vi "Drive Controller.vi"(8 "error in":errorcluster) -> ()   [LabVIEW 2018]
doc: "This VI executes continuously carrying out the current operation and responding to updates or new operation requests. It will often contain the timing or control code that is difficult to place directly in TeleOp. This VI generally opens all sensors and motors and isolates the rest of the robot code from knowing implementation details of how the operations are carried out."
uses:
  <vilib>/Rock Robotics/WPI/Framework/Completion Status.ctl
  Drive Setpoints.ctl
  Drive Operations.ctl
  Shared/RobotNeededPathData.ctl
  <vilib>/Rock Robotics/WPI/SafetyOutput/WPI_SafetyOutputConfigMenu.ctl
  <vilib>/Rock Robotics/SystemInterfaces/DIO/FPGA_DIOPWMChannel.ctl
  <vilib>/Rock Robotics/SystemInterfaces/DIO/FPGA_DIOChannel.ctl
  <vilib>/Rock Robotics/SystemInterfaces/i2clib/i2c_bus.ctl
  <vilib>/Rock Robotics/WPI/DriverStation/WPI_DriverStationRobotMode2.ctl
  <vilib>/Rock Robotics/WPI/ThirdParty/Sensors/navX/_TypeDefs/FRIC_navX_DeviceNumbersTypeDef.ctl
  <extravilib>/ChannelInstances/Lossy Stream-c(dbl,dbl,dbl,c(dbl,dbl))/Write With Abort.vi
  <extravilib>/ChannelInstances/Lossy Stream-c(dbl,dbl,dbl,c(dbl,dbl))/Read With Abort.vi
  <extravilib>/ChannelInstances/Lossy Stream-c(dbl,dbl,dbl,c(dbl,dbl))/Endpoint.vi
  <extravilib>/ChannelInstances/Lossy Stream-c(dbl,dbl,dbl,c(dbl,dbl))/EndpointRead.vi
  <vilib>/Rock Robotics/WPI/RobotDrive/WPI_RobotDriveOpen4MotorWithSPARK.vi
  <vilib>/Rock Robotics/WPI/Counter/WPI_CounterDigitalInputToDigitalSource.vi
  <vilib>/Rock Robotics/WPI/RobotDrive/WPI_RobotDriveOpen2MotorWithSPARK.vi
  Drive Published Globals.vi
  <vilib>/Rock Robotics/Network Tables/NT Write Number.vi
  <extravilib>/ChannelInstances/Lossy Stream-c(dbl,dbl,dbl,c(dbl,dbl))/Instantiate.vi
  Framework/Robot Global Data.vi
  <extravilib>/ChannelInstances/Lossy Stream-c(dbl,dbl,dbl,c(dbl,dbl))/)Channel.vi
  <resource>/ChannelSupport/_ChannelSupport/WaitIfNeeded.vi
  <vilib>/addons/control/pid/pid.llb/PID (DBL).vi
  Configuration/Constants.vi
  <vilib>/Rock Robotics/Network Tables/NT Read Number.vi
  <vilib>/addons/control/pid/NI_PID_pid.lvlib
  <extravilib>/ChannelInstances/Lossy Stream-c(dbl,dbl,dbl,c(dbl,dbl)).lvlib
panel:
  in  "Integral Range":dbl=15.0
  in  "PixyCenteringValues":cluster{"X":dbl, "Y":dbl}[](array[cluster])=[{"X"=0.0, "Y"=70.0}, {"X"=70.0, "Y"=100.0}]
  in  "EndCondArea":i32=11000
  in  "MaxY":i32=130
  in  "KpY":dbl=0.0001
  in  "KpX":dbl=0.1
  in  "MaxSpeed":dbl=0.3
  in  "KdX":dbl=0.07
  in  "AreaSetpoint":i32
  in  "CenterSetpoint":i32=80
  out "PID Tuining":cluster{dbl, dbl}(graph)={170.0, 167.02}
  in  "Points":cluster{"X":dbl, "Y":dbl}[](array[cluster])=[{"X"=0.0, "Y"=0.0}, {"X"=0.01, "Y"=0.0}, {"X"=0.011, "Y"=0.17}, {"X"=1.0, "Y"=1.0}]
  in  "PID gains":T1={"proportional gain (Kc)"=0.01, "integral time (Ti, min)"=0.007, "derivative time (Td, min)"=0.0015} {"derivative time (Td, min)" format="%#_9g"}
  out "Numeric":dbl=4.0
  out "Yaw 2":dbl=-45.089999999999996
  in  "Gains":T2={"FFV"=0.0059, "FFA"=0.0019, "Vel PID"={"P"=0.01, "I"=0.0, "D"=0.0}}
  in  "Interactive Values":T3={"Operation"=enum."Turn to Angle", "Left Speed"=-0.27, "Right Speed"=0.27, "Duration"=2.0, "Speed"=0.0, "Start Angle"=0.0, "Target Angle"=180.0, "Distance (inch)"=0.0, "Start Point (inch)"=0.0, "RobotNeededPathData"={"Path"=[], "MaxVel"=0.0, "MaxAccel"=-1.0, "Backwards?"=FALSE, "PointSpacing"=0.0, "LookaheadDist"=0.0, "Speed/Curve"=1.8, "SlowDistanceAtEnd"=12.0, "SlowSpeed"=15.0, "MaxDeAccel"=0.0}, "Start Point 2"=0.0} {"RobotNeededPathData"."SlowSpeed" format="%#_13g"; "RobotNeededPathData"."SlowDistanceAtEnd" format="%#_13g"; "RobotNeededPathData"."Speed/Curve" format="%#_13g"}
  in  "Buttons":cluster{"Execute Cmd":bool, "Abort Cmd":bool}
  out "Command Timing":cluster{"Start Time (ms)":u32, "Iterations":i32}={"Start Time (ms)"=372507, "Iterations"=0}
  out "Status":T6
  out "Setpoints":T7(graph)
  out "Current\nCmd":string="Started at  14:51:47.884\nDefault: Reserve,  L 0.0, R 0.0, D 0.000000"
  # "Tip: The graph shows the motor setpoints. It may also be helpful to observe inputs and sensor values.\nYou may also want to display tuning or debugging controls."
  # ".0088"
  # ".0017"
  # ".02"
  # "Interactive Command: You may fill in the settings for a command\nand schedule it with the Execute button. You can observe and abort\nany command while fine tuning the code for the controller."
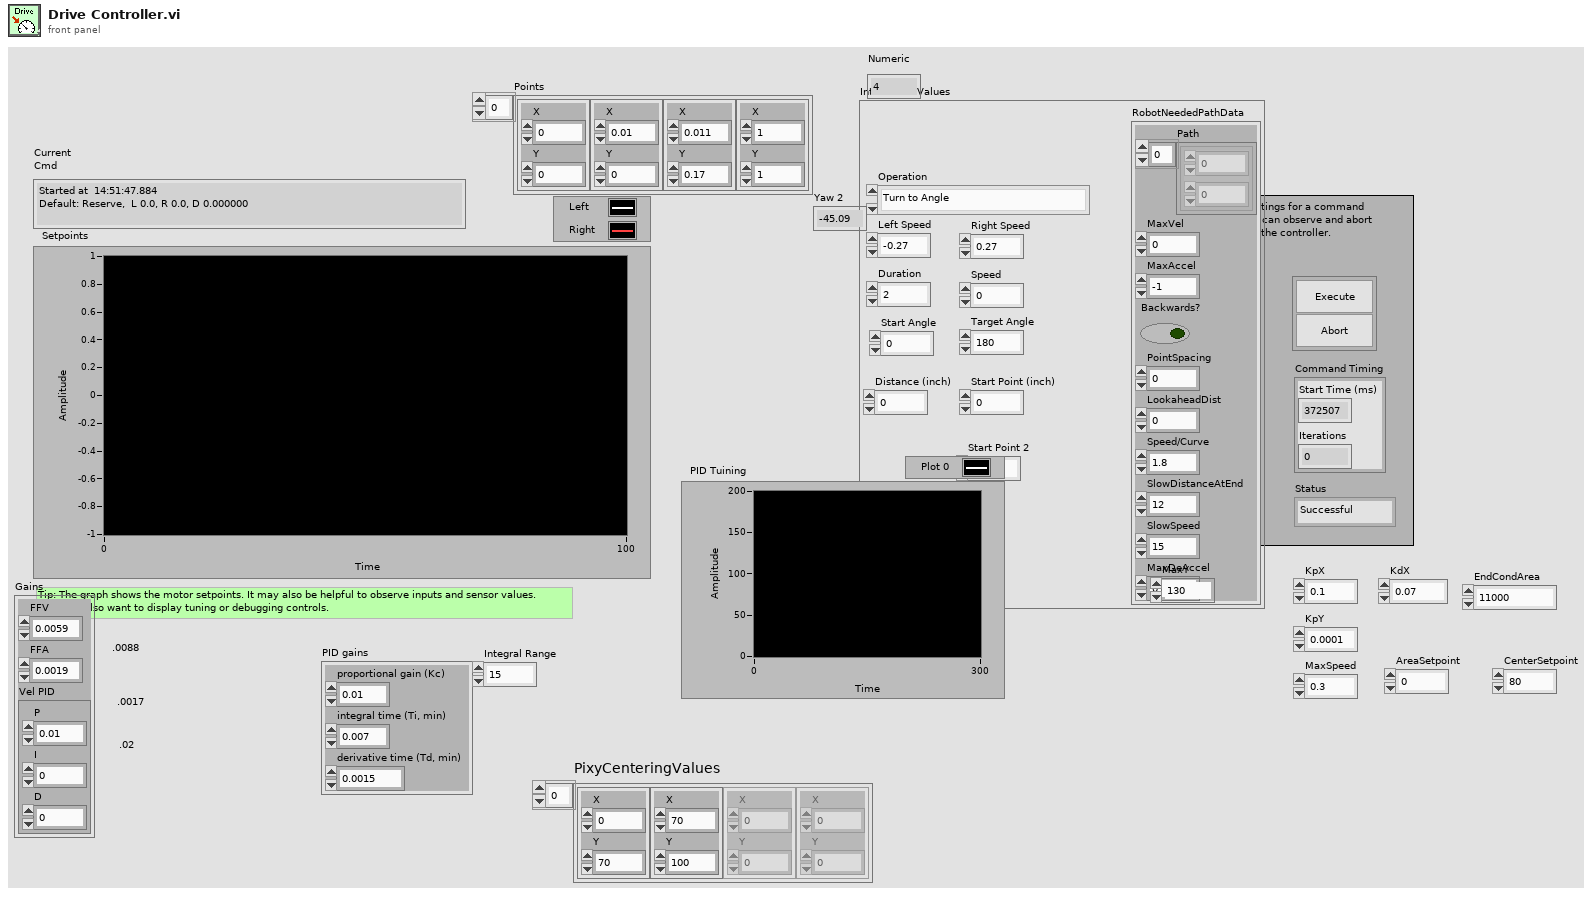
[diagram p1: front panel]
types:
  T1 = cluster{"proportional gain (Kc)":dbl, "integral time (Ti, min)":dbl, "derivative time (Td, min)":dbl}
  T2 = cluster{"FFV":dbl, "FFA":dbl, "Vel PID":cluster{"P":dbl, "I":dbl, "D":dbl}}
  T3 = typedef "Drive Setpoints.ctl" = cluster{"Operation":T4, "Left Speed":dbl, "Right Speed":dbl, "Duration":dbl, "Speed":dbl, "Start Angle":dbl, "Target Angle":dbl, "Distance (inch)":dbl, "Start Point (inch)":dbl, "RobotNeededPathData":T5, "Start Point 2":dbl}
  T4 = typedef "Drive Operations.ctl" = enum16{"Reserve", "Read Current", "Immediate", "Drive for Time", "Drive for Distance", "Turn to Angle", "Arc Turn", "Drive Path", "Drive To Cube"}
  T5 = typedef "RobotNeededPathData.ctl" = cluster{"Path":cluster{dbl, dbl}[], "MaxVel":dbl, "MaxAccel":dbl, "Backwards?":bool, "PointSpacing":dbl, "LookaheadDist":dbl, "Speed/Curve":dbl, "SlowDistanceAtEnd":dbl, "SlowSpeed":dbl, "MaxDeAccel":dbl}
  T6 = typedef "Completion Status.ctl" = enum16{"Successful", "Aborted", "Incomplete"}
  T7 = cluster{"Left Setpoint":dbl, "Right Setpoint":dbl}
  T8 = typedef "i2c_bus.ctl" = enum16{"I2C On-Board", "I2C MXP", "Invalid"}
  T9 = typedef "FPGA_DIOChannel.ctl" = enum8{"DIO 0", "DIO 1", "DIO 2", "DIO 3", "DIO 4", "DIO 5", "DIO 6", "DIO 7", "DIO 8", "DIO 9", "DIO MXP 0", "DIO MXP 1", "DIO MXP 2", "DIO MXP 3", "DIO MXP 4", "DIO MXP 5", "DIO MXP 6", "DIO MXP 7", "DIO MXP 8", "DIO MXP 9", "DIO MXP 10", "DIO MXP 11", "DIO MXP 12", "DIO MXP 13", "DIO MXP 14", "DIO MXP 15", "SPI Port CS1", "SPI Port CS2", "SPI Port CS3", "SPI Port MISO", "SPI Port MOSI", "Invalid"}
  T10 = typedef "FPGA_DIOPWMChannel.ctl" = enum8{"PWM 0", "PWM 1", "PWM 2", "PWM 3", "PWM 4", "PWM 5", "PWM 6", "PWM 7", "PWM 8", "PWM 9", "PWM MXP 0", "PWM MXP 1", "PWM MXP 2", "PWM MXP 3", "PWM MXP 4", "PWM MXP 5", "PWM MXP 6", "PWM MXP 7", "PWM MXP 8", "PWM MXP 9", "Invalid"}
  T11 = typedef "WPI_SafetyOutputConfigMenu.ctl" = enum16{"Enable", "Disable"}
  T12 = typedef "WPI_DigitalInputDevRef.ctl" = cluster{"DevStatus":errorcluster, "DIO Channel":T9}
  T13 = typedef "FPGA_CounterEncoderSourceConvertionLVSourceType.ctl" = cluster{"DevStatus":errorcluster, "AnalogTriggerMode?":bool, "DigitalMode":cluster{"DIO Channel":T14}, "AnalogTriggerMode":cluster{"AnalogTriggerIndex":T15, "OutputType":T16}}
  T14 = typedef "FPGA_DIODigitalSourceChannel.ctl" = enum8{"DIO 0", "DIO 1", "DIO 2", "DIO 3", "DIO 4", "DIO 5", "DIO 6", "DIO 7", "DIO 8", "DIO 9", "DIO MXP 0", "DIO MXP 1", "DIO MXP 2", "DIO MXP 3", "DIO MXP 4", "DIO MXP 5", "DIO MXP 6", "DIO MXP 7", "DIO MXP 8", "DIO MXP 9", "DIO MXP 10", "DIO MXP 11", "DIO MXP 12", "DIO MXP 13", "DIO MXP 14", "DIO MXP 15", "SPI Port CS1", "SPI Port CS2", "SPI Port CS3", "SPI Port MISO", "SPI Port MOSI", "Disabled"}
  T15 = typedef "FPGA_AnalogTriggerIndex.ctl" = enum8{"Trig 0", "Trig 1", "Trig 2", "Trig 3", "Trig 4", "Trig 5", "Trig 6", "Trig 7", "Invalid"}
  T16 = typedef "FPGA_AnalogTriggerOutType.ctl" = enum16{"InWindow", "TriggerState", "Rising", "Falling"}
  T17 = typedef "WPI_EncoderDevRef.ctl" = cluster{"DevStatus":errorcluster, "EncoderIndex":T18, "CounterIndex":T19, "DistancePerCount":dbl, "Decoding Type":T20}
  T18 = typedef "FPGA_EncoderIdx.ctl" = enum8{"Enc 0", "Enc 1", "Enc 2", "Enc 3", "Enc 4", "Enc 5", "Enc 6", "Enc 7", "Invalid"}
  T19 = typedef "FPGA_CounterCtrSystemIndex.ctl" = enum8{"Ctr 0", "Ctr 1", "Ctr 2", "Ctr 3", "Ctr 4", "Ctr 5", "Ctr 6", "Ctr 7", "Invalid"}
  T20 = typedef "WPI_EncoderType.ctl" = enum16{"1x", "2x", "4x"}
  T21 = typedef "WPI_RobotDriveDevRef.ctl" = cluster{"DevStatus":errorcluster, "Motors[]":T22[], "Square Inputs":bool, "Max Output":dbl}
  T22 = typedef "WPI_MotorControlDeviceRef.ctl" = cluster{"DeviceStatus":errorcluster, "Type":T23, "PWM":cluster{"PWM Channel":T10, "DeadBand":T24}, "CAN":cluster{"Device Number":u8, "SetOutput VI Ref":variant, "GetOutput VI Ref":variant, "Enable VI Ref":variant, "Disable VI Ref":variant, "Data":variant}, "Invert":bool, "DIO PWM":cluster{"PWM \"Enable\" Channel":T10, "DIOChannel":T9, "PWM Rate":dbl}}
  T23 = typedef "WPI_MotorControlType.ctl" = enum16{"PWM", "CAN", "DIO PWM"}
  T24 = typedef "WPI_PWMDeadband.ctl" = cluster{"Name":string, "maxPositivePwm":i32, "minPositivePwm":i32, "centerPwm":i32, "maxNegativePwm":i32, "minNegativePwm":i32, "angularRange":u16}
  T25 = typedef "Command Status Info.ctl" = cluster{"Name":string, "Status":T6, "notifier out":T26}
  T26 = typedef "Completion Notifier.ctl" = refnum<notifier>
  T27 = cluster{"SubSystem Data":T3, cluster{"Start Time (ms)":u32, "Iterations":i32}, cluster{"Command Info":T25, "Description":string, "Default Command":T3, "queue out":refnum<queue>, "Subsystem Name":string}}
  T28 = typedef "WPI_I2CDevRef.ctl" = cluster{"DevStatus":errorcluster, "Device Address":u8, "Handle":i32, "I2C Bus":T8}
  T29 = cluster{"X":i32, "Y":i32, "Width":i32, "Height":i32, "ValidData":bool, "Timestamp":u32}
  T30 = typedef "WPI_DriverStationRobotMode2.ctl" = enum16{"Autonomous Disabled", "Autonomous Enabled", "Teleop Disabled", "Teleop Enabled", "Disconnected", "Finish", "Test Disabled", "Test Enabled", "Emergency Stopped"}
  T31 = cluster{"Yaw":dbl, "Roll":dbl, "Pitch":dbl, "Heading":dbl, "Fused Heading":dbl}
  T32 = cluster{"dx/dt":dbl, "dx/dt":dbl, dbl, cluster{dbl, dbl}}
  T33 = typedef "Lossy Stream-c(dbl,dbl,dbl,c(dbl,dbl)).lvlib/)Channel.ctl" = refnum<queue>
  T34 = typedef "FRIC_navX_DeviceNumbersTypeDef.ctl" = enum16{"Dev0", "Dev1", "Dev2", "Dev3"}
  T35 = cluster{"LeftDistance":dbl, "RightDistance":dbl, "LeftVelocity":dbl, "RightVelocity":dbl, "Angle":dbl, "Location":cluster{dbl, dbl}}
  T36 = cluster{"dx/dt":dbl, "dx/dt":dbl, "Yaw":dbl, cluster{dbl, dbl}}
  T37 = cluster{"SubSystem Data":T3, cluster{"Start Time (ms)":u32, "Iterations":i32}, "Default Command Arguments":cluster{"Command Info":T25, "Description":string, "Default Command":T3, "queue out":refnum<queue>, "Subsystem Name":string}}
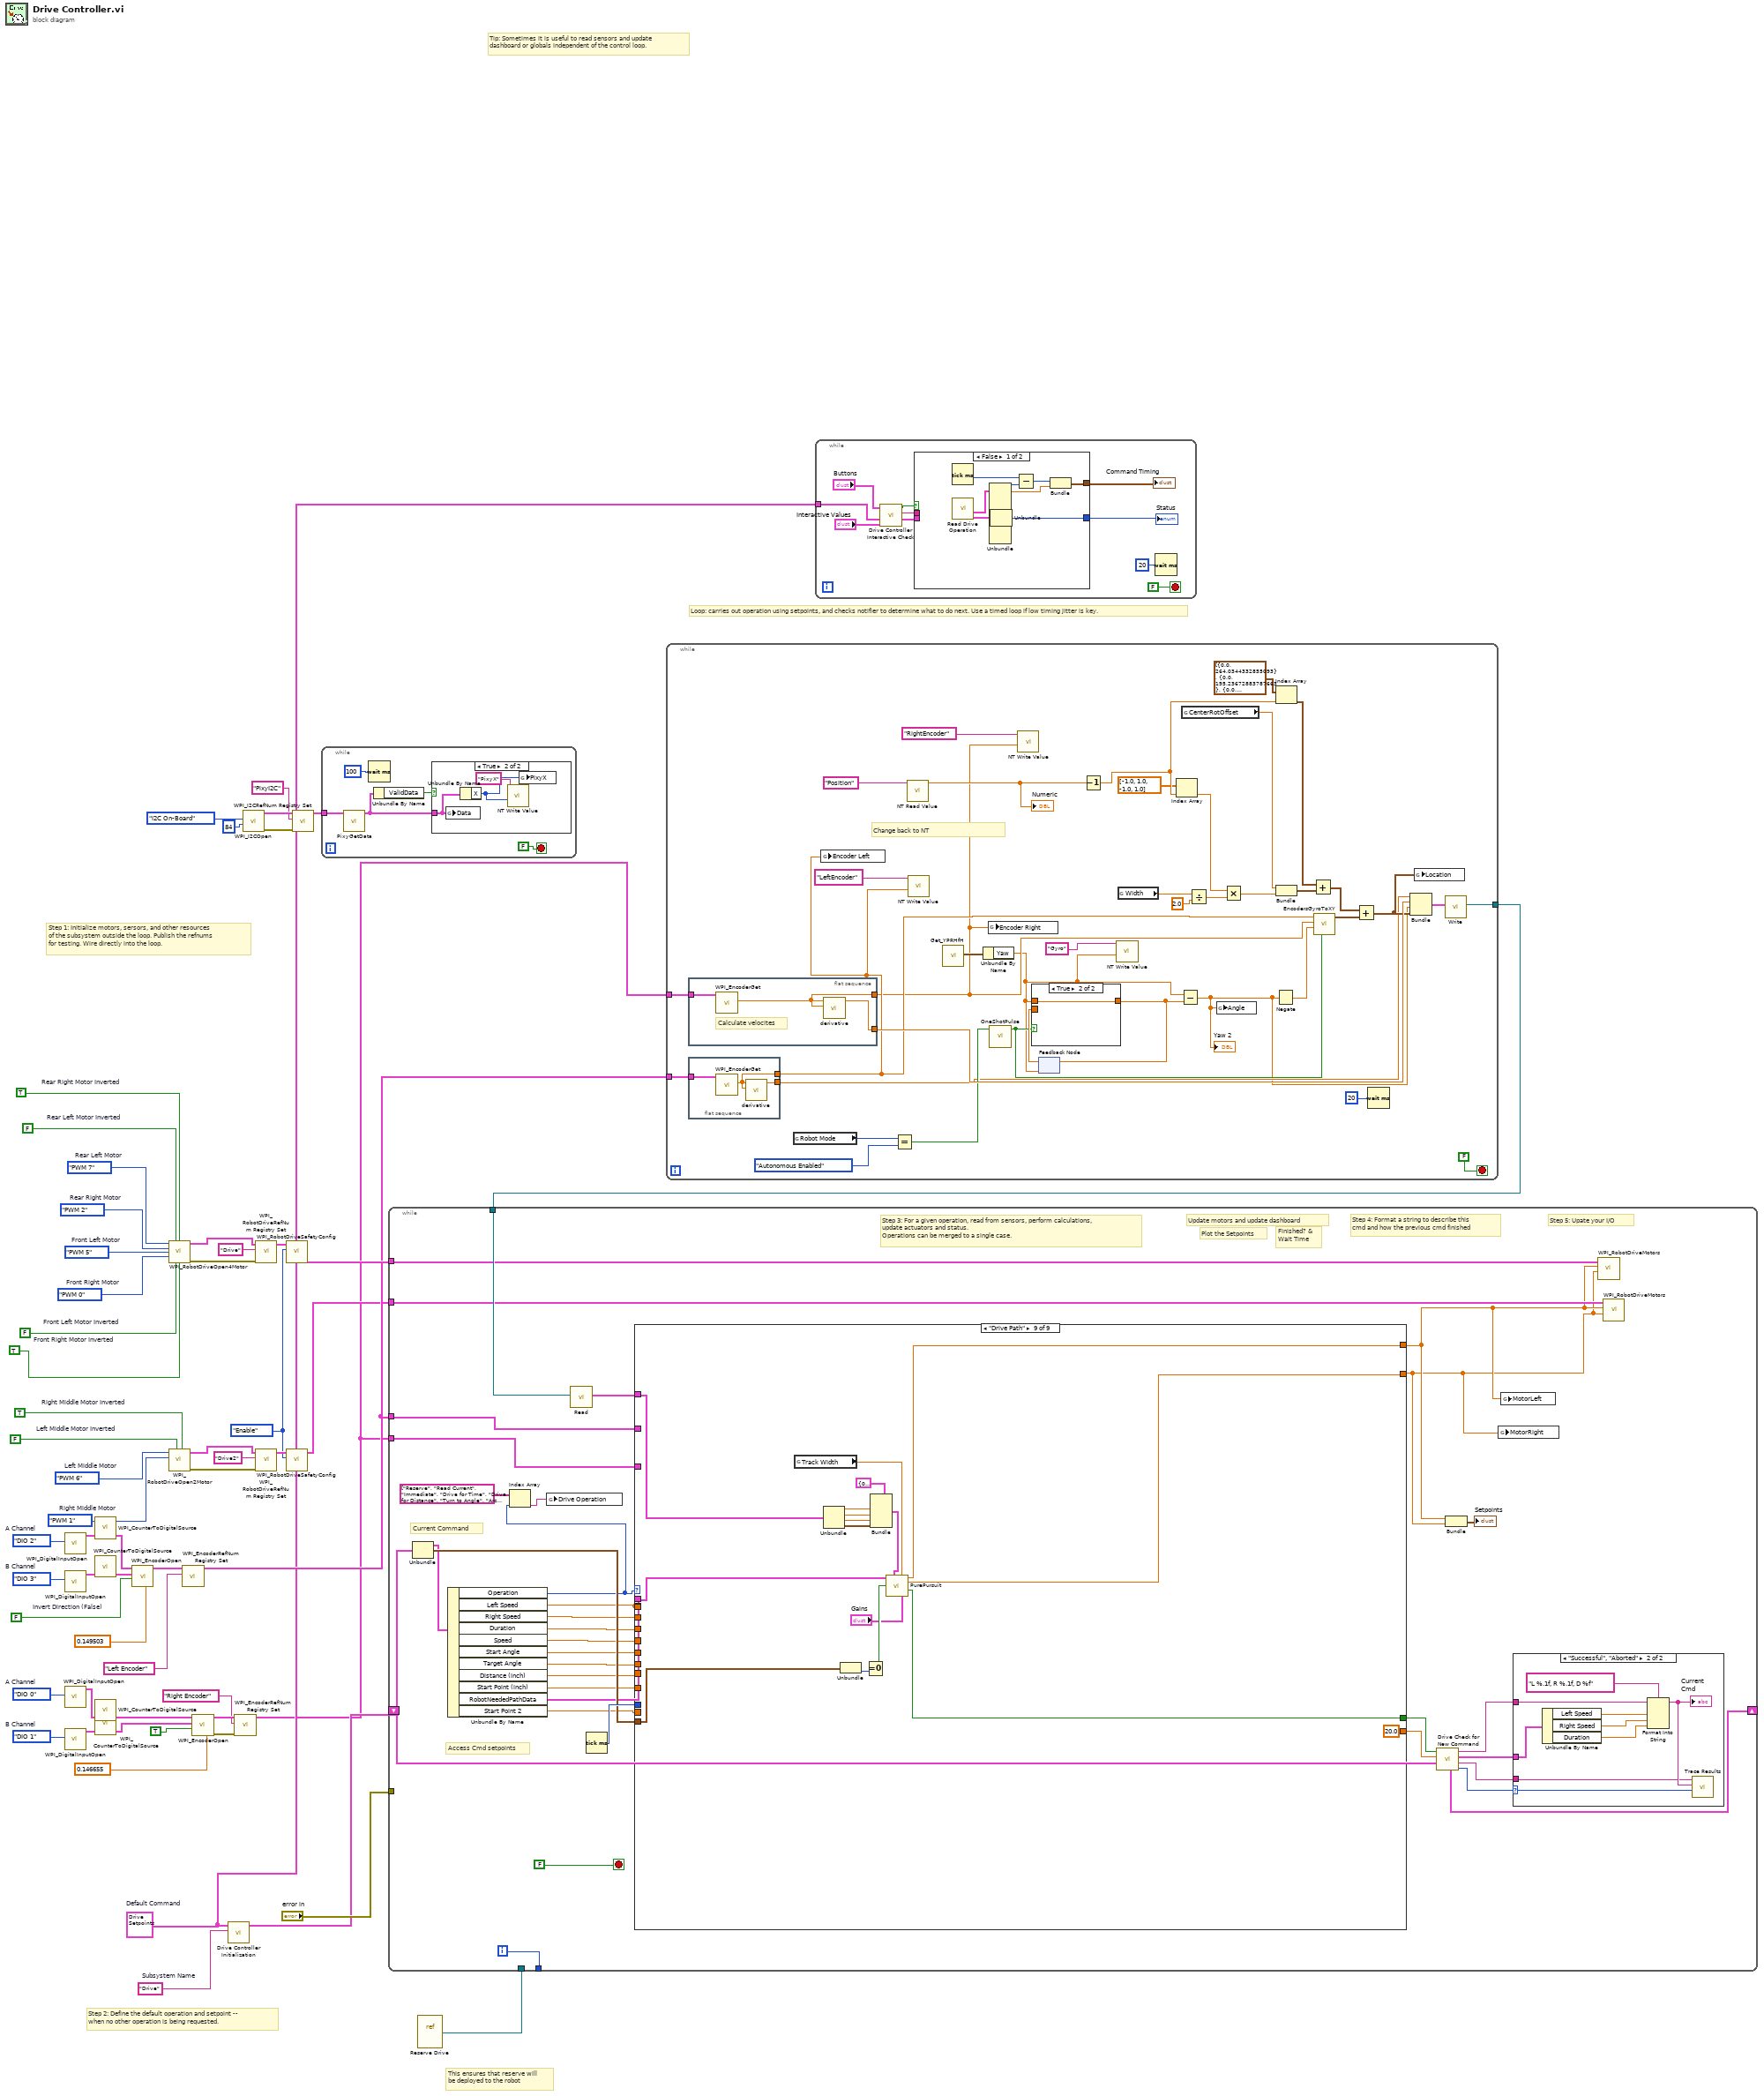
[diagram p0: block diagram]
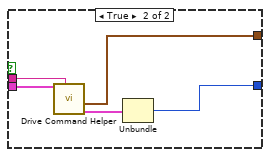
[diagram p4: hidden frame]
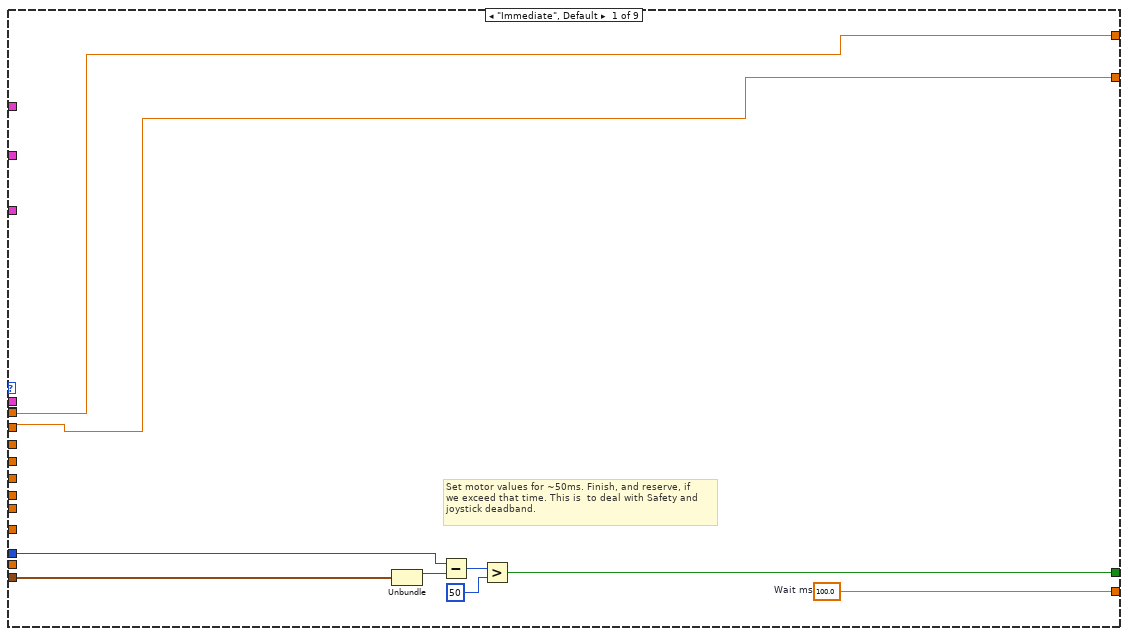
[diagram p5: hidden frame]
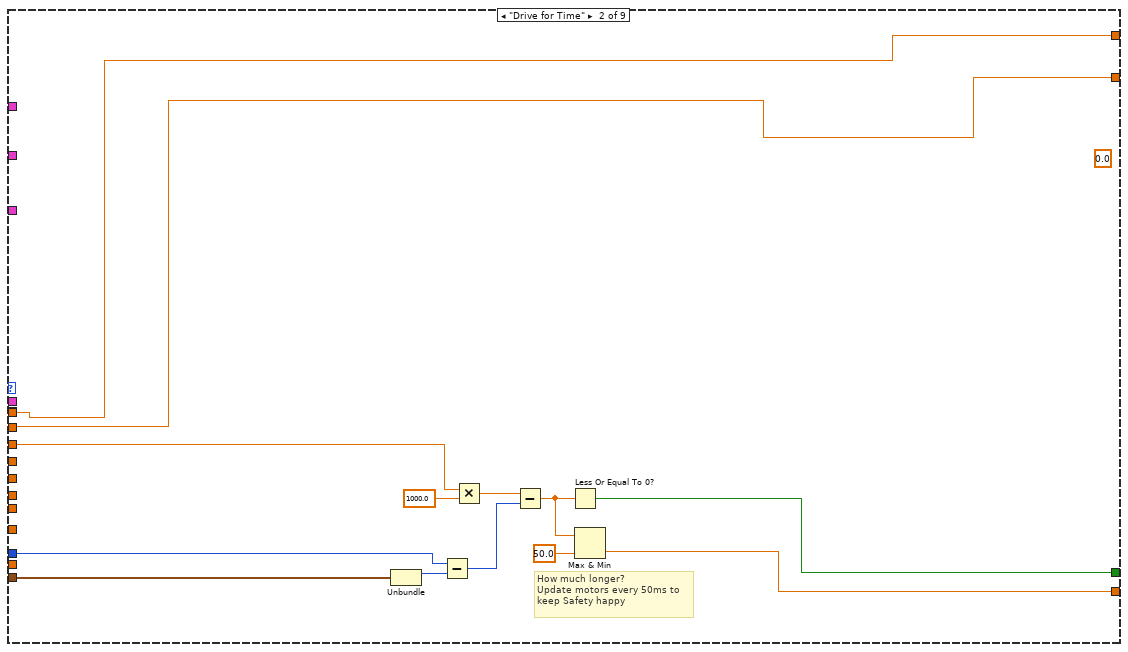
[diagram p6: hidden frame]
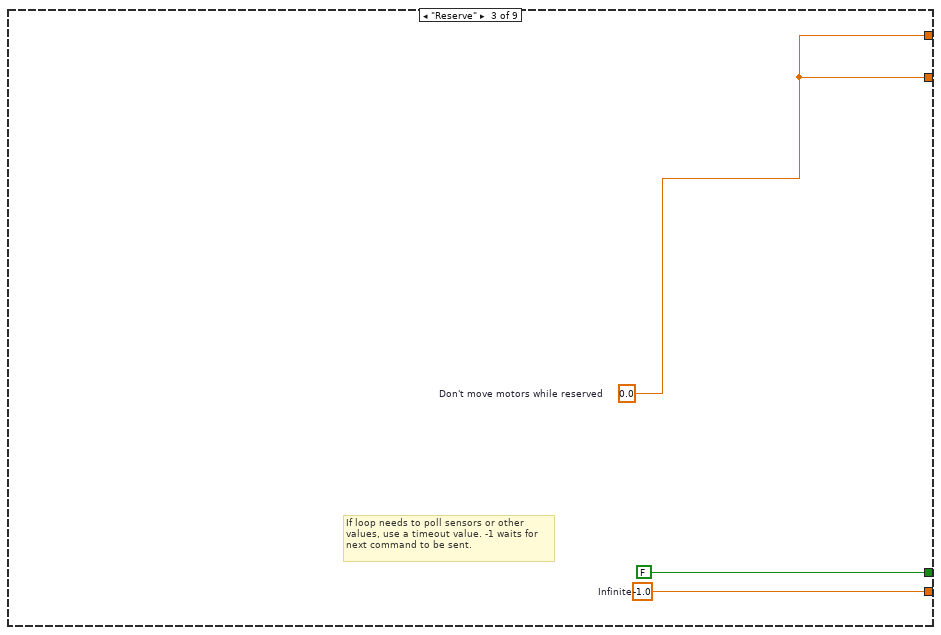
[diagram p7: hidden frame]
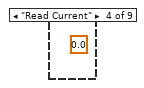
[diagram p8: hidden frame]
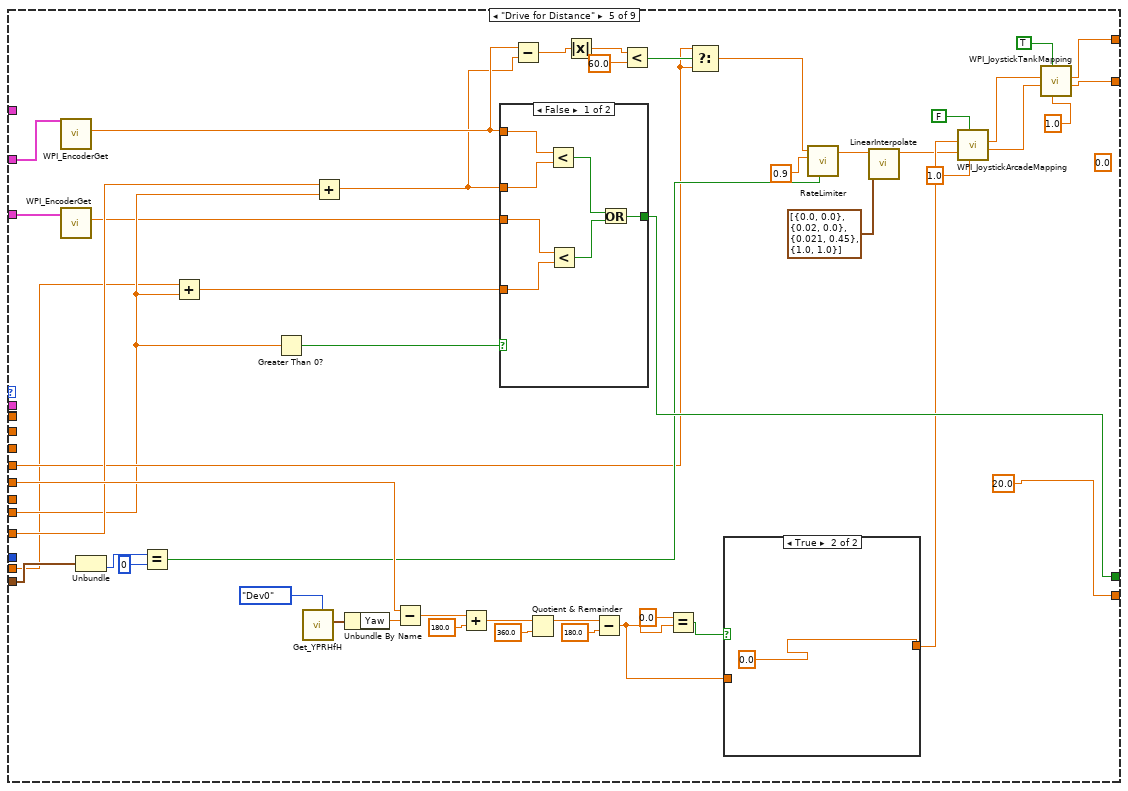
[diagram p9: hidden frame]
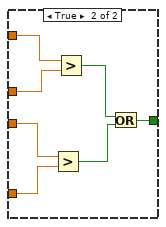
[diagram p10: hidden frame]
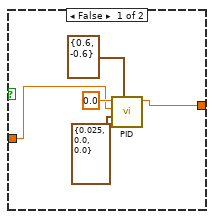
[diagram p11: hidden frame]
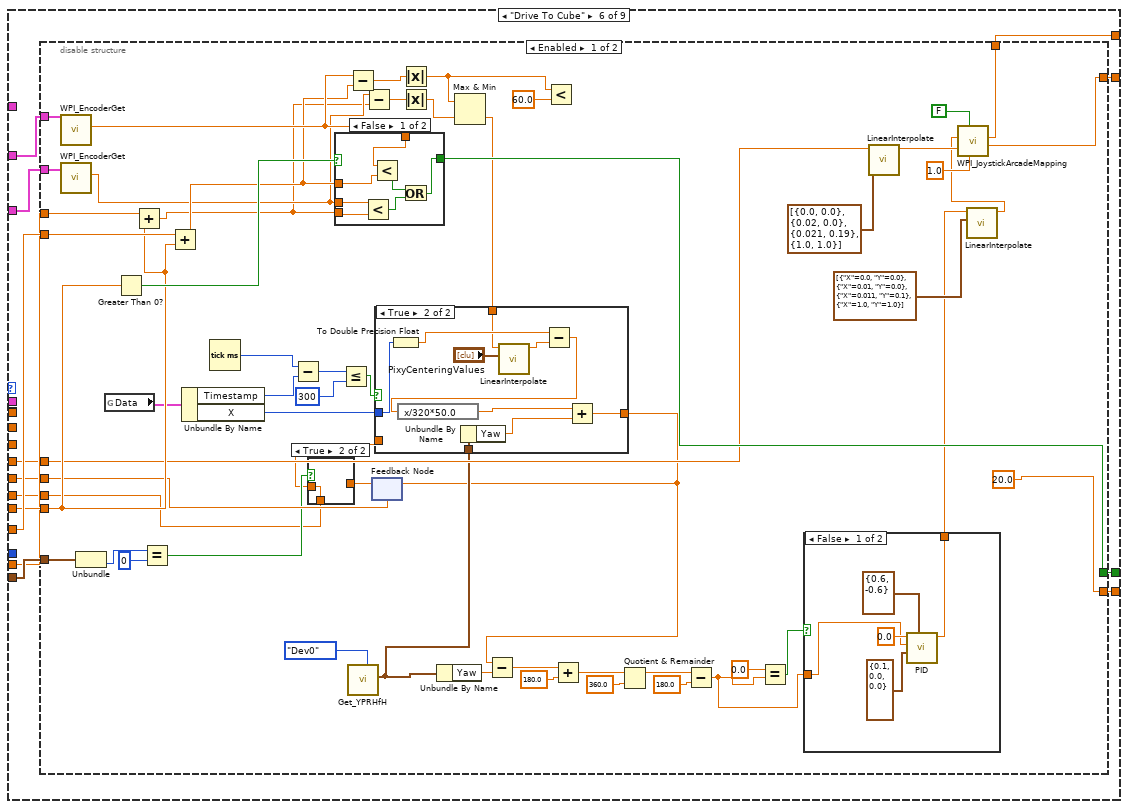
[diagram p12: hidden frame]
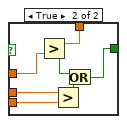
[diagram p15: hidden frame]
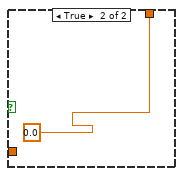
[diagram p16: hidden frame]
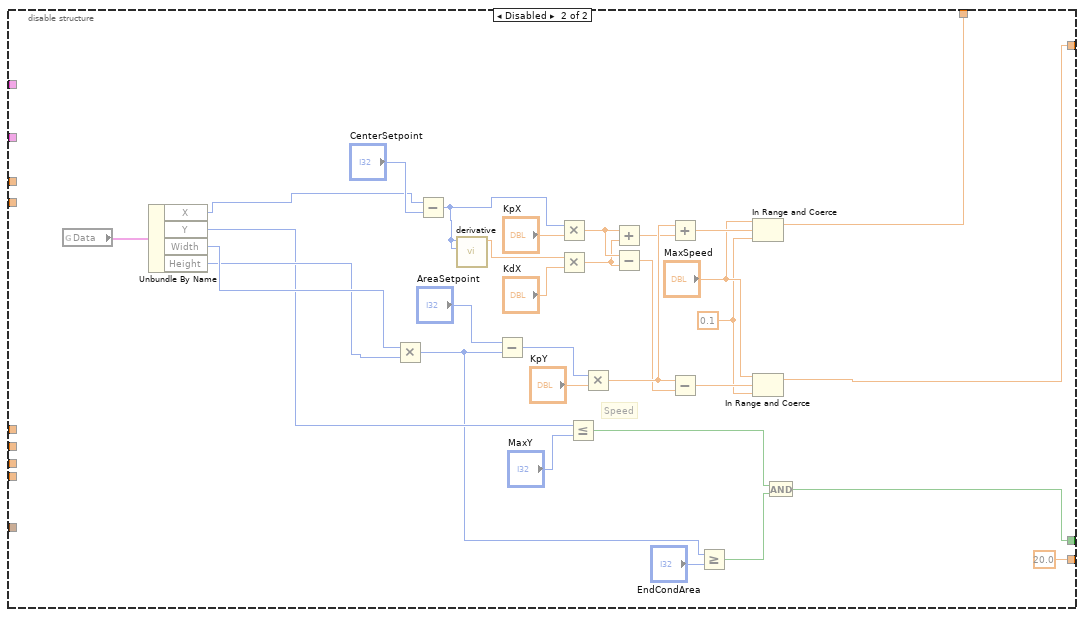
[diagram p17: hidden frame]
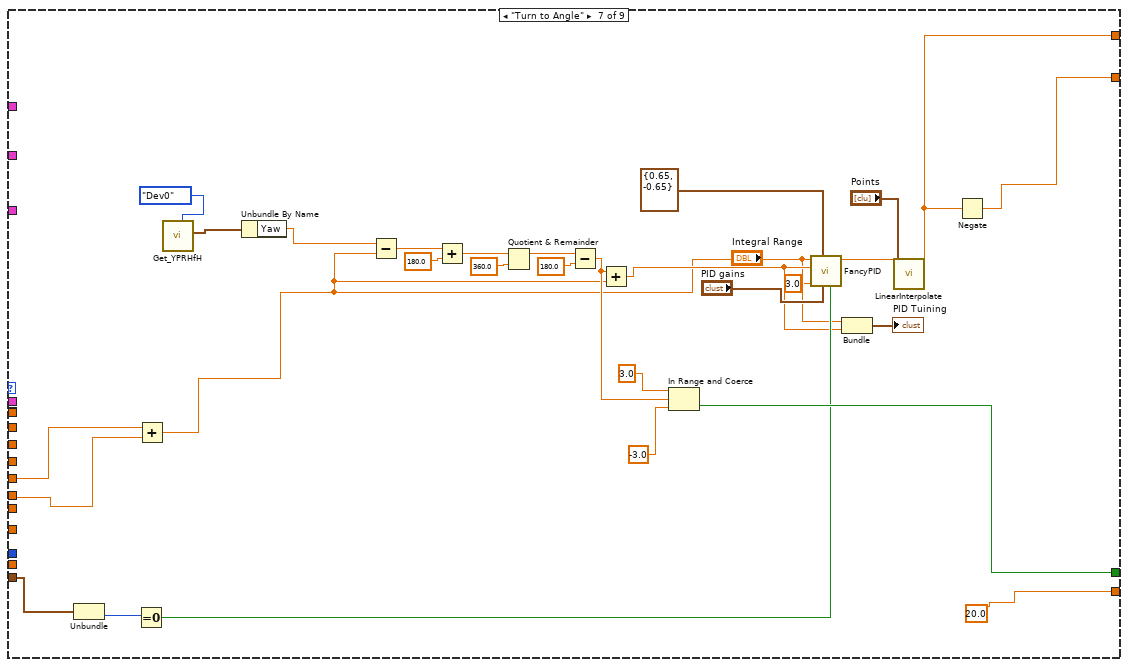
[diagram p18: hidden frame]
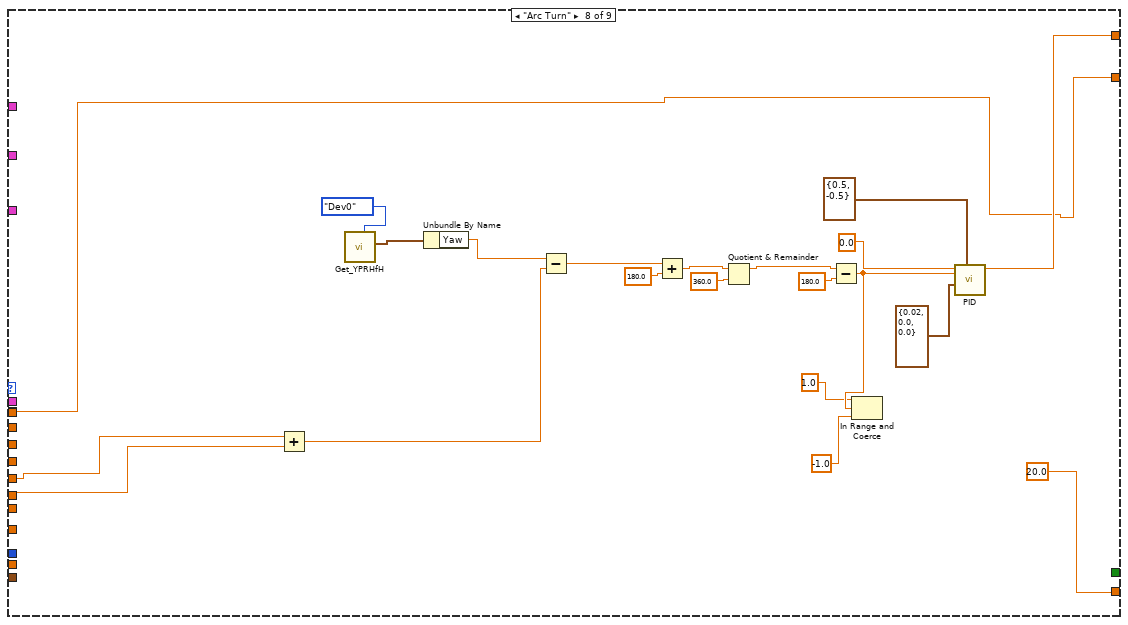
[diagram p19: hidden frame]
diagram:
  w10 = FPGA_DIOChannel."DIO 1"  # B Channel
  w13 = FPGA_DIOChannel."DIO 0"  # A Channel
  w20 = T3 {"Operation"=enum."Reserve", "Left Speed"=0.0, "Right Speed"=0.0, "Duration"=0.0, "Speed"=0.0, "Start Angle"=0.0, "Target Angle"=0.0, "Distance (inch)"=0.0, "Start Point (inch)"=0.0, "RobotNeededPathData"={"Path"=[], "MaxVel"=0.0, "MaxAccel"=0.0, "Backwards?"=FALSE, "PointSpacing"=0.0, "LookaheadDist"=0.0, "Speed/Curve"=1.8, "SlowDistanceAtEnd"=12.0, "SlowSpeed"=15.0, "MaxDeAccel"=0.0}, "Start Point 2"=0.0}  # Default Command
  w27 = TRUE  # Right Middle Motor Inverted
  w28 = FALSE  # Left Middle Motor Inverted
  w31 = FPGA_DIOPWMChannel."PWM 1"  # Right Middle Motor
  w32 = FPGA_DIOPWMChannel."PWM 6"  # Left Middle Motor
  w41 = FALSE  # Invert Direction (False)
  w34 = FPGA_DIOChannel."DIO 3"  # B Channel
  w35 = FPGA_DIOChannel."DIO 2"  # A Channel
  w43 = TRUE  # Front Right Motor Inverted
  w44 = FALSE  # Front Left Motor Inverted
  w45 = TRUE  # Rear Right Motor Inverted
  w46 = FALSE  # Rear Left Motor Inverted
  w47 = FPGA_DIOPWMChannel."PWM 0"  # Front Right Motor
  w48 = FPGA_DIOPWMChannel."PWM 5"  # Front Left Motor
  w49 = FPGA_DIOPWMChannel."PWM 2"  # Rear Right Motor
  w50 = FPGA_DIOPWMChannel."PWM 7"  # Rear Left Motor
  w22 = WPI_SafetyOutputConfigMenu."Enable" ("mode")
  w58 = "Drive"  # Subsystem Name
  # "Step 1: Initialize motors, sersors, and other resources\nof the subsystem outside the loop. Publish the refnums\nfor testing. Wire directly into the loop."
  # "Step 2: Define the default operation and setpoint --\nwhen no other operation is being requested."
  # "This ensures that reserve will\nbe deployed to the robot"
  # "Tip: Sometimes it is useful to read sensors and update\ndashboard or globals independent of the control loop."
  # "Loop: carries out operation using setpoints, and checks notifier to determine what to do next. Use a timed loop if low timing jitter is key."
  n1 = call <vilib>:"WPI_DigitalInputOpen.vi"("DIO Channel"=w35) -> ("DigitalInputDevRef"=w38:T12)  [unwired: 1 in, 9 out]
  n2 = call <vilib>:"WPI_DigitalInputOpen.vi"("DIO Channel"=w34) -> ("DigitalInputDevRef"=w37:T12)  [unwired: 1 in, 9 out]
  n3 = call <vilib>:"WPI_DigitalInputOpen.vi"("DIO Channel"=w13) -> ("DigitalInputDevRef"=w14:T12)  [unwired: 1 in, 9 out]
  n4 = call <vilib>:"WPI_DigitalInputOpen.vi"("DIO Channel"=w10) -> ("DigitalInputDevRef"=w11:T12)  [unwired: 1 in, 9 out]
  n5 = call-poly <vilib>:"WPI_CounterToDigitalSource.vi"("DigitalInputDevRef"=w38) -> ("Digital Source"=w39:T13)  [unwired: 6 out]
  n6 = call-poly <vilib>:"WPI_CounterToDigitalSource.vi"("DigitalInputDevRef"=w37) -> ("Digital Source"=w36:T13)  [unwired: 6 out]
  n7 = call-poly <vilib>:"WPI_CounterToDigitalSource.vi"("DigitalInputDevRef"=w14) -> ("Digital Source"=w15:T13)  [unwired: 6 out]
  n8 = call-poly <vilib>:"WPI_CounterToDigitalSource.vi"("DigitalInputDevRef"=w11) -> ("Digital Source"=w12:T13)  [unwired: 6 out]
  n9 = call <vilib>:"WPI_EncoderOpen.vi"("DistancePerCount"=0.149503, "Invert Direction (False)"=w41, "BSource"=w36, "ASource"=w39) -> ("EncoderDevRef"=w40:T17)  [unwired: 4 in, 3 out]
  n10 = call-poly <vilib>:"WPI_RobotDriveOpen4Motor.vi"("Rear Left Motor"=w50, "Rear Left Motor Inverted"=w46, "Rear Right Motor Inverted"=w45, "Rear Right Motor"=w49, "Front Left Motor"=w48, "Front Right Motor"=w47, "Front Left Motor Inverted"=w44, "Front Right Motor Inverted"=w43) -> ("RobotDriveDevRef"=w57:T21, "error out"=w55:errorcluster)  [unwired: 6 in]
  n11 = call-poly <vilib>:"WPI_RobotDriveOpen2Motor.vi"("Right Motor Inverted"=w27, "Left Motor Inverted"=w28, "Right Motor"=w31, "Left Motor"=w32) -> ("error out"=w26:errorcluster, "RobotDriveDevRef"=w30:T21)  [unwired: 6 in]
  n12 = call <vilib>:"WPI_EncoderRefNum Registry Set.vi"("refnum name"="Left Encoder", "EncoderDevRef"=w40) -> ("EncoderDevRef"=w33:T17)  [unwired: 8 in, 1 out]
  n13 = call <vilib>:"WPI_EncoderOpen.vi"("DistancePerCount"=0.146655, "Invert Direction (False)"=TRUE, "BSource"=w12, "ASource"=w15) -> ("error out"=w17:errorcluster, "EncoderDevRef"=w16:T17)  [unwired: 4 in, 2 out]
  n14 = call "Drive Controller Initialization.vi"("Subsystem Name"=w58, "Default Command"=w20) -> ("Current Command"=w52:T27)  [unwired: 9 in]
  n15 = call <vilib>:"WPI_EncoderRefNum Registry Set.vi"("error in (no error)"=w17, "refnum name"="Right Encoder", "EncoderDevRef"=w16) -> ("EncoderDevRef"=w18:T17)  [unwired: 7 in, 1 out]
  n16 = call <vilib>:"WPI_I2COpen.vi"("Device Address"=u8 84, "I2C Bus"=i2c_bus."I2C On-Board") -> ("error out"=w3:errorcluster, "I2CDevRef"=w4:T28)  [unwired: 8 in]
  n17 = call <vilib>:"WPI_RobotDriveRefNum Registry Set.vi"("error in (no error)"=w55, "refnum name"="Drive", "RobotDriveDevRef"=w57) -> ("RobotDriveDevRef"=w25:T21)  [unwired: 1 in, 7 out]
  n18 = call <vilib>:"WPI_RobotDriveRefNum Registry Set.vi"("error in (no error)"=w26, "refnum name"="Drive2", "RobotDriveDevRef"=w30) -> ("RobotDriveDevRef"=w24:T21)  [unwired: 7 in, 1 out]
  n19 = call <vilib>:"WPI_RobotDriveSafetyConfig.vi"("mode"=w22, "RobotDriveDevRef"=w25) -> ("RobotDriveDevRef"=w54:T21)  [unwired: 8 in, 1 out]
  n20 = call <vilib>:"WPI_RobotDriveSafetyConfig.vi"("mode"=w22, "RobotDriveDevRef"=w24) -> ("RobotDriveDevRef"=w23:T21)  [unwired: 8 in, 1 out]
  n21 = call <vilib>:"WPI_I2CRefNum Registry Set.vi"("error in (no error)"=w3, "refnum name"="PixyI2C", "I2CDevRef"=w4) -> ("I2CDevRef"=w1:T28)  [unwired: 7 in, 1 out]
  n22 = while {
    tunnel: w1 -> [w62]
    stop <- FALSE stop-if-true
    n23 = call "PixyGetData.vi"("I2CDevRef"=w62) -> ("Data"=w61:T29)  [unwired: 10 in]
    n24 = Wait (ms)(milliseconds to wait=u32 100) -> ()  [unwired: 1 out]
    n25 = Unbundle By Name(w61) -> ("ValidData"=w60:bool)
    n26 = case shown="True" w60 {
      tunnel: w61 -> [_ w66]
      frame False {
      }
      frame True {
        n27 = global write "Drive Published Globals.vi" "Data"(w66) -> ()
        n28 = Unbundle By Name(w66) -> ("X"=w64:i32)
        n29 = call-poly <vilib>:"NT Write Value.vi"("Numeric"=w64, "Name"="PixyX") -> ()  [unwired: 9 in, 1 out]
        n30 = global write "Drive Published Globals.vi" "PixyX"(w64) -> ()
      }
    }
  }
  n31 = vi-ref "Reserve Drive.vi"() -> (w51:refnum<vi>)
  n32 = while {
    tunnel: [w78] -> w19
    tunnel: w18 -> [w77]
    tunnel: w33 -> [w76]
    stop <- FALSE stop-if-true
    # "Change back to NT"
    n33 = flat-sequence {
      tunnel: [w112] -> w102
      tunnel: [w111] -> w68
      tunnel: w77 -> [w113]
      frame #0 {
        # "Calculate velocites"
        n34 = call <vilib>:"WPI_EncoderGet.vi"("EncoderDevRef"=w113) -> ("Distance"=w111:dbl)  [unwired: 5 in, 5 out]
        n35 = call "derivative.vi"("Starting value"=w111, "x"=w111) -> ("dx/dt"=w112:dbl)  [unwired: 9 in]
      }
    }
    n36 = flat-sequence {
      tunnel: [w108] -> w79
      tunnel: [w107] -> w70
      tunnel: w76 -> [w106]
      frame #0 {
        n37 = call <vilib>:"WPI_EncoderGet.vi"("EncoderDevRef"=w106) -> ("Distance"=w107:dbl)  [unwired: 5 in, 5 out]
        n38 = call "derivative.vi"("Starting value"=w107, "x"=w107) -> ("dx/dt"=w108:dbl)  [unwired: 9 in]
      }
    }
    n39 = global read "Robot Global Data.vi" "Robot Mode"() -> (w93:T30)
    n40 = global write "Drive Published Globals.vi" "Encoder Left"(w70) -> ()
    n41 = Equal?(x=w93, y=WPI_DriverStationRobotMode2."Autonomous Enabled") -> (x = y?=w94:bool)
    n42 = call-poly <vilib>:"NT Read Value.vi"("Name"="Position") -> ("Numeric"=w74:dbl)  [unwired: 9 in, 1 out]
    "Numeric" <- w74
    n43 = call-poly <vilib>:"NT Write Value.vi"("Numeric"=w70, "Name"="LeftEncoder") -> ()  [unwired: 9 in, 1 out]
    n44 = call <vilib>:"Get_YPRHfH.vi"() -> ("YRPHfH"=w105:T31)  [unwired: 11 in]
    n45 = Unbundle By Name(w105) -> ("Yaw"=w67:dbl)
    n46 = global write "Drive Published Globals.vi" "Encoder Right"(w68) -> ()
    n47 = call "OneShotPulse.vi"("Input"=w94) -> ("Output"=w95:bool)  [unwired: 10 in]
    n48 = call-poly <vilib>:"NT Write Value.vi"("Numeric"=w68, "Name"="RightEncoder") -> ()  [unwired: 9 in, 1 out]
    n49 = feedback #1(w67) -> (w96:dbl)
    n50 = case shown="True" w95 {
      tunnel: w67 -> [_ w110]
      tunnel: [w109 w110] -> w97
      tunnel: w96 -> [w109 _]
      frame False {
      }
      frame True {
      }
    }
    n51 = feedback-in #1(w97) -> ()
    n52 = Decrement(x=w74) -> (x-1=w87:dbl)
    n53 = call-poly <vilib>:"NT Write Value.vi"("Numeric"=w67, "Name"="Gyro") -> ()  [unwired: 9 in, 1 out]
    n54 = global read "Constants.vi" "Width"() -> (w82:dbl)
    n55 = Index Array(array=dbl[] [-1.0, 1.0, -1.0, 1.0], index=w87) -> (element=w88:dbl)
    n56 = Subtract(x=w67, y=w97) -> (x-y=w72:dbl)
    "Yaw 2" <- w72
    n57 = global read "Constants.vi" "CenterRotOffset"() -> (w80:dbl)
    n58 = Divide(x=w82, y=2.0) -> (x/y=w83:dbl)
    n59 = global write "Drive Published Globals.vi" "Angle"(w72) -> ()
    n60 = Multiply(x=w88, y=w83) -> (x*y=w89:dbl)
    n61 = Negate(x=w72) -> (-x=w98:dbl)
    n62 = Index Array(array=cluster{dbl, dbl}[] [{0.0, 264.0344332855093}, {0.0, 195.23672883787663}, {0.0, 144.10329985652797}, {0.0, -0.0}] ("x*y"), index=w87) -> (element=w86:cluster{dbl, dbl})
    n63 = Bundle("CenterRotOffset"=w80, w89) -> (w90:cluster{"CenterRotOffset":dbl, dbl})  [unwired: 1 in]
    n64 = Add(x=w86, y=w90) -> (x+y=w91:cluster{dbl, dbl})
    n65 = call "EncodersGyroToXY.vi"("Reset"=w95, "Angle (degrees)"=w98, "Right Distance"=w68, "Left Distance"=w70) -> ("Location"=w99:cluster{dbl, dbl})  [unwired: 7 in]
    n66 = Add(x=w91, y=w99) -> (x+y=w100:cluster{dbl, dbl})
    n67 = Wait (ms)(milliseconds to wait=u32 20) -> ()  [unwired: 1 out]
    n68 = Bundle("dx/dt"=w79, "dx/dt"=w102, w72, w100) -> (w101:T32)  [unwired: 1 in]
    n69 = global write "Drive Published Globals.vi" "Location"(w100) -> ()
    n70 = call <extravilib>:"Write.vi"("element"=w101) -> ("channel"=w78:T33)  [unwired: 8 in, 2 out]
  }
  n71 = while {
    shift-right: [w144] -> _
    shift-left: w52 -> [w114]
    tunnel: [w147] -> _
    tunnel: w54 -> [w124]
    tunnel: "error in" -> [_]
    tunnel: w51 -> [_]
    tunnel: w33 -> [w122]
    tunnel: w23 -> [w123]
    tunnel: w19 -> [w126]
    tunnel: w18 -> [w121]
    i -> [w147]
    stop <- FALSE stop-if-true
    # "Plot the Setpoints"
    # "Step 5: Upate your I/O"
    # "Step 4: Format a string to describe this\ncmd and how the previous cmd finished"
    # "Current Command"
    # "Update motors and update dashboard"
    # "Access Cmd setpoints"
    # "Finished? &\nWait Time"
    # "Step 3: For a given operation, read from sensors, perform calculations,\nupdate actuators and status.\nOperations can be merged to a single case."
    n72 = Unbundle(w114) -> ("SubSystem Data"=w127:T3, w138:cluster{"Start Time (ms)":u32, "Iterations":i32})  [unwired: 1 out]
    n73 = Unbundle By Name(w127) -> ("Operation"=w117:T4, "Left Speed"=w136:dbl, "Right Speed"=w135:dbl, "Duration"=w134:dbl, "Speed"=w133:dbl, "Start Angle"=w132:dbl, "Target Angle"=w131:dbl, "Distance (inch)"=w130:dbl, "Start Point (inch)"=w129:dbl, "RobotNeededPathData"=w128:T5, "Start Point 2"=w120:dbl)
    n74 = Index Array(array=string[] ["Reserve", "Read Current", "Immediate", "Drive for Time", "Drive for Distance", "Turn to Angle", "Arc Turn", "Drive Path", "Drive To Cube"] ("Strings []"), index=w117) -> (element=w115:string)
    n75 = global write "Robot Global Data.vi" "Drive Operation"(w115) -> ()
    n76 = call <extravilib>:"Read.vi"("channel"=w126) -> ("element"=w125:T36)  [unwired: 5 in, 5 out]
    n77 = Tick Count (ms)() -> (millisecond timer value=w146:u32)
    n78 = case shown="\"Drive Path\"" w117 {
      tunnel: [w157 w161 w173 _ 20.0 ("Infinite") w253 20.0 ("Infinite") 20.0 ("Infinite") 20.0 ("Infinite")] -> w143
      tunnel: [w152 w165 FALSE ("ignore previous (F)") _ w209 w254 w397 _ w439] -> w142
      tunnel: w138 -> [w151 w167 _ _ w190 w250 w387 _ w429]
      tunnel: w146 -> [w153 w164 _ _ _ _ _ _ _]
      tunnel: [w150 w159 w171 _ w195 w245 w385 w406 w441] -> w119
      tunnel: [w149 w158 w171 _ w196 w244 w384 w405 w440] -> w118
      tunnel: w133 -> [_ _ _ _ w179 w246 _ _ _]
      tunnel: w130 -> [_ _ _ _ w177 w248 _ _ _]
      tunnel: w134 -> [_ w160 _ _ _ _ _ _ _]
      tunnel: w136 -> [w150 _ _ _ _ _ _ w405 _]
      tunnel: w135 -> [w149 w158 _ _ _ _ _ _ _]
      tunnel: w122 -> [_ _ _ _ w207 w252 _ _ _]
      tunnel: w132 -> [_ _ _ _ w203 w243 w400 w409 _]
      tunnel: w131 -> [_ _ _ _ _ w242 w399 w408 _]
      tunnel: w129 -> [_ _ _ _ w202 w251 _ _ _]
      tunnel: w136 -> [_ w159 _ _ _ _ _ _ _]
      tunnel: w128 -> [_ _ _ _ _ _ _ _ w442]
      tunnel: w125 -> [_ _ _ _ _ _ _ _ w433]
      tunnel: w121 -> [_ _ _ _ w178 w249 _ _ _]
      tunnel: w120 -> [_ _ _ _ w176 w247 _ _ _]
      frame "Immediate", Default {
        w157 = 100.0  # Wait ms
        # "Set motor values for ~50ms. Finish, and reserve, if\nwe exceed that time. This is  to deal with Safety and\njoystick deadband."
        n79 = Unbundle(w151) -> ("Start Time (ms)"=w154:u32)  [unwired: 1 out]
        n80 = Subtract(x=w153, y=w154) -> (x-y=w155:u32)
        n81 = Greater?(x=w155, y=u8 50 ("Left Motor")) -> (0:w152:bool)
      }
      frame "Drive for Time" {
        (unwired) 0.0 ("output")
        # "How much longer?\nUpdate motors every 50ms to\nkeep Safety happy"
        n82 = Unbundle(w167) -> ("Start Time (ms)"=w166:u32)  [unwired: 1 out]
        n83 = Subtract(x=w164, y=w166) -> (x-y=w170:u32)
        n84 = Multiply(x=w160, y=1000.0) -> (x*y=w169:dbl)
        n85 = Subtract(x=w169, y=w170) -> (x-y=w163:dbl)
        n86 = Less Or Equal To 0?(x=w163) -> (x <= 0?=w165:bool)
        n87 = Max & Min(x=w163, y=50.0) -> (min(x,y)=w161:dbl)  [unwired: 1 out]
      }
      frame "Reserve" {
        w171 = 0.0  # Don't move motors while reserved
        w173 = -1.0  # Infinite
        # "If loop needs to poll sensors or other\nvalues, use a timeout value. -1 waits for\nnext command to be sent."
      }
      frame "Read Current" {
        (unwired) 0.0 ("output")
      }
      frame "Drive for Distance" {
        (unwired) 0.0 ("output")
        n88 = call <vilib>:"WPI_EncoderGet.vi"("EncoderDevRef"=w207) -> ("Distance"=w186:dbl)  [unwired: 5 in, 5 out]
        n89 = call <vilib>:"WPI_EncoderGet.vi"("EncoderDevRef"=w178) -> ("Distance"=w174:dbl)  [unwired: 5 in, 5 out]
        n90 = Unbundle(w190) -> ("Iterations"=w189:i32)  [unwired: 1 out]
        n91 = Equal?(x=w189, y=0) -> (x = y?=w187:bool)
        n92 = Add(x=w176, y=w177) -> (x+y=w175:dbl)
        n93 = Greater Than 0?(x=w177) -> (x > 0?=w201:bool)
        n94 = call <vilib>:"Get_YPRHfH.vi"("Device Number"=FRIC_navX_DeviceNumbersTypeDef."Dev0") -> ("YRPHfH"=w221:T31)  [unwired: 10 in]
        n95 = Add(x=w202, y=w177) -> (x+y=w185:dbl)
        n96 = Unbundle By Name(w221) -> ("Yaw"=w212:dbl)
        n97 = Subtract(x=w203, y=w212) -> (x-y=w211:dbl)
        n98 = Add(x=w211, y=180.0) -> (x+y=w216:dbl)
        n99 = case shown="False" w201 {
          tunnel: w186 -> [w227 w235]
          tunnel: w185 -> [w228 w234]
          tunnel: [w225 w229] -> w209
          tunnel: w175 -> [w223 w233]
          tunnel: w174 -> [w224 w232]
          frame False {
            n100 = Less?(x=w227, y=w228) -> (x < y?=w226:bool)
            n101 = Less?(x=w224, y=w223) -> (x < y?=w222:bool)
            n102 = Or(x=w226, y=w222) -> (x .or. y?=w225:bool)
          }
          frame True {
            n103 = Greater?(x=w232, y=w233) -> (0:w230:bool)
            n104 = Greater?(x=w235, y=w234) -> (0:w231:bool)
            n105 = Or(x=w231, y=w230) -> (x .or. y?=w229:bool)
          }
        }
        n106 = Subtract(x=w186, y=w185) -> (x-y=w184:dbl)
        n107 = Quotient & Remainder(x=w216, y=360.0) -> (x-y*floor(x/y)=w214:dbl)  [unwired: 1 out]
        n108 = Absolute Value(x=w184) -> (abs(x)=w183:dbl)
        n109 = Subtract(x=w214, y=180.0) -> (x-y=w210:dbl)
        n110 = Less?(x=w183, y=60.0) -> (x < y?=w181:bool)
        n111 = Equal?(x=0.0, y=w210) -> (x = y?=w219:bool)
        n112 = Select(t=w179, s=w181, f=w179) -> (s? t:f=w180:dbl)
        n113 = case shown="True" w219 {
          tunnel: [w236 0.0] -> w204
          tunnel: w210 -> [w237 _]
          frame False {
            n114 = call-poly <vilib>:"PID.vi"("output range"=cluster{"output high":dbl, "output low":dbl} {"output high"=0.6, "output low"=-0.6}, "PID gains"=T1 {"proportional gain (Kc)"=0.025, "integral time (Ti, min)"=0.0, "derivative time (Td, min)"=0.0}, "process variable"=w237, "setpoint"=0.0) -> ("output"=w236:dbl)  [unwired: 6 in, 1 out]
          }
          frame True {
          }
        }
        n115 = call "RateLimiter.vi"("Reset"=w187, "Max dx/dt"=0.9, "Input"=w180) -> ("Output"=w198:dbl)  [unwired: 8 in]
        n116 = call "LinearInterpolate.vi"("Points"=cluster{"X":dbl, "Y":dbl}[] [{"X"=0.0, "Y"=0.0}, {"X"=0.02, "Y"=0.0}, {"X"=0.021, "Y"=0.45}, {"X"=1.0, "Y"=1.0}], "Value"=w198) -> ("Output"=w199:dbl)  [unwired: 9 in]
        n117 = call <vilib>:"WPI_JoystickArcadeMapping.vi"("Max Output"=1.0, "Square Inputs"=FALSE, "Y axis value"=w199, "X axis value"=w204) -> ("Right Motor Value"=w194:dbl, "Left Motor Value"=w193:dbl)  [unwired: 6 in]
        n118 = call <vilib>:"WPI_JoystickTankMapping.vi"("Max Output"=1.0, "Square Inputs"=TRUE, "Right axis value"=w194, "Left axis value"=w193) -> ("Right Motor Value"=w196:dbl, "Left Motor Value"=w195:dbl)  [unwired: 6 in]
      }
      frame "Drive To Cube" {
        n119 = disable-structure shown="Enabled" {
          disable-tunnel: [w300 w344] -> w254
          disable-tunnel: [20.0 ("Infinite") 20.0 ("Infinite")] -> w253
          disable-tunnel: w252 -> [w298 _]
          disable-tunnel: w251 -> [w295 _]
          disable-tunnel: w250 -> [w291 _]
          disable-tunnel: w249 -> [w284 _]
          disable-tunnel: w248 -> [w283 _]
          disable-tunnel: w247 -> [w282 _]
          disable-tunnel: w246 -> [w281 _]
          disable-tunnel: [w280 w358] -> w245
          disable-tunnel: [w279 w359] -> w244
          disable-tunnel: w243 -> [w275 _]
          disable-tunnel: w242 -> [w270 _]
          frame Enabled {
            n120 = call <vilib>:"WPI_EncoderGet.vi"("EncoderDevRef"=w298) -> ("Distance"=w288:dbl)  [unwired: 5 in, 5 out]
            n121 = call <vilib>:"WPI_EncoderGet.vi"("EncoderDevRef"=w284) -> ("Distance"=w261:dbl)  [unwired: 5 in, 5 out]
            n122 = Unbundle(w291) -> ("Iterations"=w290:i32)  [unwired: 1 out]
            n123 = global read "Drive Published Globals.vi" "Data"() -> (w278:T29)
            n124 = Greater Than 0?(x=w283) -> (x > 0?=w294:bool)
            n125 = Add(x=w282, y=w283) -> (x+y=w260:dbl)
            n126 = Equal?(x=w290, y=0) -> (x = y?=w273:bool)
            n127 = Add(x=w295, y=w283) -> (x+y=w287:dbl)
            n128 = Unbundle By Name(w278) -> ("Timestamp"=w266:u32, "X"=w277:i32)
            n129 = Tick Count (ms)() -> (millisecond timer value=w265:u32)
            n130 = Subtract(x=w265, y=w266) -> (x-y=w264:u32)
            n131 = case shown="False" w294 {
              tunnel: w288 -> [w329 w337]
              tunnel: w287 -> [w330 w336]
              tunnel: [w327 w331] -> w300
              tunnel: w260 -> [w325 w335]
              tunnel: w261 -> [w326 w334]
              frame False {
                n132 = Less?(x=w326, y=w325) -> (x < y?=w324:bool)
                n133 = Less?(x=w329, y=w330) -> (x < y?=w328:bool)
                n134 = Or(x=w328, y=w324) -> (x .or. y?=w327:bool)
              }
              frame True {
                n135 = Greater?(x=w337, y=w336) -> (0:w333:bool)
                n136 = Greater?(x=w334, y=w335) -> (0:w332:bool)
                n137 = Or(x=w333, y=w332) -> (x .or. y?=w331:bool)
              }
            }
            n138 = Less Or Equal?(x=w264, y=u32 300) -> (x <= y?=w262:bool)
            n139 = Subtract(x=w288, y=w287) -> (x-y=w286:dbl)
            n140 = call <vilib>:"Get_YPRHfH.vi"("Device Number"=FRIC_navX_DeviceNumbersTypeDef."Dev0") -> ("YRPHfH"=w276:T31)  [unwired: 10 in]
            n141 = Subtract(x=w261, y=w260) -> (x-y=w259:dbl)
            n142 = feedback #2(w275) -> (w271:dbl)
            n143 = case shown="True" w273 {
              tunnel: [w311 w312] -> w272
              tunnel: w271 -> [w311 _]
              tunnel: w270 -> [_ w312]
              frame False {
              }
              frame True {
              }
            }
            n144 = Absolute Value(x=w286) -> (abs(x)=w258:dbl)
            n145 = Absolute Value(x=w259) -> (abs(x)=w257:dbl)
            n146 = Unbundle By Name(w276) -> ("Yaw"=w302:dbl)
            n147 = Max & Min(x=w258, y=w257) -> (min(x,y)=w256:dbl)  [unwired: 1 out]
            n148 = case shown="True" w262 {
              tunnel: w277 -> [_ w319]
              tunnel: w272 -> [w313 _]
              tunnel: w276 -> [_ w321]
              tunnel: [w313 w320] -> w274
              tunnel: w256 -> [_ w314]
              frame False {
              }
              frame True {
                n149 = To Double Precision Float(number=w319) -> (double precision float=w318:dbl)
                n150 = Unbundle By Name(w321) -> ("Yaw"=w322:dbl)
                n151 = call "LinearInterpolate.vi"("Points"="PixyCenteringValues", "Value"=w314) -> ("Output"=w317:dbl)  [unwired: 9 in]
                n152 = Subtract(x=w318, y=w317) -> (x-y=w316:dbl)
                n153 = expression code="x/320*50.0"(w316) -> (w323:dbl)
                n154 = Add(x=w323, y=w322) -> (x+y=w320:dbl)
              }
            }
            n155 = feedback-in #2(w274) -> ()
            n156 = Subtract(x=w274, y=w302) -> (x-y=w301:dbl)
            n157 = Less?(x=w258, y=60.0) -> ()  [unwired: 1 out]
            n158 = Add(x=w301, y=180.0) -> (x+y=w306:dbl)
            n159 = Quotient & Remainder(x=w306, y=360.0) -> (x-y*floor(x/y)=w304:dbl)  [unwired: 1 out]
            n160 = Subtract(x=w304, y=180.0) -> (x-y=w255:dbl)
            n161 = Equal?(x=0.0, y=w255) -> (x = y?=w309:bool)
            n162 = case shown="False" w309 {
              tunnel: [w338 0.0] -> w268
              tunnel: w255 -> [w339 _]
              frame False {
                n163 = call-poly <vilib>:"PID.vi"("output range"=cluster{"output high":dbl, "output low":dbl} {"output high"=0.6, "output low"=-0.6}, "PID gains"=T1 {"proportional gain (Kc)"=0.1, "integral time (Ti, min)"=0.0, "derivative time (Td, min)"=0.0}, "process variable"=w339, "setpoint"=0.0) -> ("output"=w338:dbl)  [unwired: 6 in, 1 out]
              }
              frame True {
              }
            }
            n164 = call "LinearInterpolate.vi"("Points"=cluster{"X":dbl, "Y":dbl}[] [{"X"=0.0, "Y"=0.0}, {"X"=0.02, "Y"=0.0}, {"X"=0.021, "Y"=0.19}, {"X"=1.0, "Y"=1.0}], "Value"=w281) -> ("Output"=w293:dbl)  [unwired: 9 in]
            n165 = call "LinearInterpolate.vi"("Points"=cluster{"X":dbl, "Y":dbl}[] [{"X"=0.0, "Y"=0.0}, {"X"=0.01, "Y"=0.0}, {"X"=0.011, "Y"=0.1}, {"X"=1.0, "Y"=1.0}], "Value"=w268) -> ("Output"=w267:dbl)  [unwired: 9 in]
            n166 = call <vilib>:"WPI_JoystickArcadeMapping.vi"("Max Output"=1.0, "Square Inputs"=FALSE, "Y axis value"=w293, "X axis value"=w267) -> ("Right Motor Value"=w279:dbl, "Left Motor Value"=w280:dbl)  [unwired: 6 in]
          }
          frame Disabled {
            w362 = 0.1 ("lower limit")
            # "Speed"
            n167 = global read "Drive Published Globals.vi" "Data"() -> (w357:T29)
            n168 = Unbundle By Name(w357) -> ("X"=w356:i32, "Y"=w348:i32, "Width"=w353:i32, "Height"=w352:i32)
            n169 = Multiply(x=w353, y=w352) -> (x*y=w347:i32)
            n170 = Subtract(x=w356, y="CenterSetpoint") -> (x-y=w355:i32)
            n171 = call "derivative.vi"("Starting value"=w355, "x"=w355) -> ("dx/dt"=w354:dbl)  [unwired: 9 in]
            n172 = Subtract(x="AreaSetpoint", y=w347) -> (x-y=w369:i32)
            n173 = Multiply(x=w355, y="KpX") -> (x*y=w366:dbl)
            n174 = Multiply(x=w354, y="KdX") -> (x*y=w365:dbl)
            n175 = Less Or Equal?(x=w348, y="MaxY") -> (x <= y?=w345:bool)
            n176 = Multiply(x=w369, y="KpY") -> (x*y=w370:dbl)
            n177 = Add(x=w366, y=w365) -> (x+y=w367:dbl)
            n178 = Subtract(x=w366, y=w365) -> (x-y=w364:dbl)
            n179 = Add(x=w370, y=w367) -> (x+y=w372:dbl)
            n180 = Subtract(x=w370, y=w364) -> (x-y=w371:dbl)
            n181 = Greater Or Equal?(x=w347, y="EndCondArea") -> (x >= y?=w346:bool)
            n182 = In Range and Coerce(upper limit="MaxSpeed", x=w372, lower limit=w362) -> (coerced(x)=w358:dbl)  [unwired: 1 out]
            n183 = In Range and Coerce(upper limit="MaxSpeed", x=w371, lower limit=w362) -> (coerced(x)=w359:dbl)  [unwired: 1 out]
            n184 = And(x=w345, y=w346) -> (x .and. y?=w344:bool)
          }
        }
      }
      frame "Turn to Angle" {
        n185 = Unbundle(w387) -> ("Iterations"=w386:i32)  [unwired: 1 out]
        n186 = Equal To 0?(x=w386) -> (x = 0?=w380:bool)
        n187 = Add(x=w400, y=w399) -> (x+y=w377:dbl)
        n188 = call <vilib>:"Get_YPRHfH.vi"("Device Number"=FRIC_navX_DeviceNumbersTypeDef."Dev0") -> ("YRPHfH"=w402:T31)  [unwired: 10 in]
        n189 = Unbundle By Name(w402) -> ("Yaw"=w390:dbl)
        n190 = Subtract(x=w390, y=w377) -> (x-y=w391:dbl)
        n191 = Add(x=w391, y=180.0) -> (x+y=w394:dbl)
        n192 = Quotient & Remainder(x=w394, y=360.0) -> (x-y*floor(x/y)=w392:dbl)  [unwired: 1 out]
        n193 = Subtract(x=w392, y=180.0) -> (x-y=w389:dbl)
        n194 = Add(x=w389, y=w377) -> (x+y=w378:dbl)
        n195 = In Range and Coerce(upper limit=3.0, x=w389, lower limit=-3.0) -> (In Range?=w397:bool)  [unwired: 1 out]
        n196 = call "FancyPID.vi"("Reset"=w380, "Gains"="PID gains", "Range"=cluster{"output high":dbl, "output low":dbl} {"output high"=0.65, "output low"=-0.65} ("output range"), "Disable Range"=3.0, "Integral Range"="Integral Range", "Process variable"=w378, "Setpoint"=w377) -> ("output"=w381:dbl)  [unwired: 4 in]
        n197 = Bundle(w377, w378) -> (→"PID Tuining":cluster{dbl, dbl})  [unwired: 1 in]
        n198 = call "LinearInterpolate.vi"("Points"="Points", "Value"=w381) -> ("Output"=w385:dbl)  [unwired: 9 in]
        n199 = Negate(x=w385) -> (-x=w384:dbl)
      }
      frame "Arc Turn" {
        n200 = Add(x=w409, y=w408) -> (x+y=w416:dbl)
        n201 = call <vilib>:"Get_YPRHfH.vi"("Device Number"=FRIC_navX_DeviceNumbersTypeDef."Dev0") -> ("YRPHfH"=w412:T31)  [unwired: 10 in]
        n202 = Unbundle By Name(w412) -> ("Yaw"=w410:dbl)
        n203 = Subtract(x=w410, y=w416) -> (x-y=w418:dbl)
        n204 = Add(x=w418, y=180.0) -> (x+y=w421:dbl)
        n205 = Quotient & Remainder(x=w421, y=360.0) -> (x-y*floor(x/y)=w419:dbl)  [unwired: 1 out]
        n206 = Subtract(x=w419, y=180.0) -> (x-y=w415:dbl)
        n207 = In Range and Coerce(upper limit=1.0, x=w415, lower limit=-1.0) -> ()  [unwired: 2 out]
        n208 = call-poly <vilib>:"PID.vi"("output range"=cluster{"output high":dbl, "output low":dbl} {"output high"=0.5, "output low"=-0.5}, "PID gains"=T1 {"proportional gain (Kc)"=0.02, "integral time (Ti, min)"=0.0, "derivative time (Td, min)"=0.0}, "process variable"=w415, "setpoint"=0.0) -> ("output"=w406:dbl)  [unwired: 6 in, 1 out]
      }
      frame "Drive Path" {
        n209 = global read "Constants.vi" "Track Width"() -> (w428:dbl)
        n210 = Unbundle(w433) -> ("dx/dt"=w437:dbl, "dx/dt"=w436:dbl, "Yaw"=w435:dbl, w434:cluster{dbl, dbl})
        n211 = Unbundle(w429) -> ("Iterations"=w430:i32)  [unwired: 1 out]
        n212 = Equal To 0?(x=w430) -> (x = 0?=w431:bool)
        n213 = Bundle(cluster=T35 {"LeftDistance"=0.0, "RightDistance"=0.0, "LeftVelocity"=0.0, "RightVelocity"=0.0, "Angle"=0.0, "Location"={0.0, 0.0}} ("SensorData"), "LeftVelocity"=w437, "RightVelocity"=w436, "Angle"=w435, "Location"=w434) -> (w438:T35)  [unwired: 2 in]
        n214 = call "PurePursuit.vi"("RobotNeededPathData"=w442, "SensorData"=w438, "Trackwidth"=w428, "Reset"=w431, "Gains"="Gains") -> ("LeftValue"=w441:dbl, "RightValue"=w440:dbl, "Done"=w439:bool)  [unwired: 6 in, 2 out]
      }
    }
    n215 = call "Drive Check for New Command.vi"("input cluster"=w114, "Wait time (ms)"=w143, "Finished?"=w142) -> ("Completion"=w145:T6, "Subsystem Name"=w139:string, "Current Command"=w140:T3, "Initial Trace String"=w141:string, "Next Command"=w144:T37)  [unwired: 4 in]
    n216 = Bundle("LeftValue"=w119, "RightValue"=w118) -> (→"Setpoints":cluster{"LeftValue":dbl, "RightValue":dbl})  [unwired: 1 in]
    n217 = global write "Drive Published Globals.vi" "MotorRight"(w118) -> ()
    n218 = global write "Drive Published Globals.vi" "MotorLeft"(w119) -> ()
    n219 = case shown="\"Successful\", \"Aborted\"" w145 {
      selector: w145 -> [_ w451]
      tunnel: w141 -> [_ w446]
      tunnel: w140 -> [_ w447]
      tunnel: w139 -> [_ w443]
      frame "Incomplete", Default {
        # "Continuing current command"
      }
      frame "Successful", "Aborted" {
        # "Report and setup for next command"
        n220 = Unbundle By Name(w447) -> ("Left Speed"=w449:dbl, "Right Speed"=w450:dbl, "Duration"=w444:dbl)
        n221 = Format Into String(format string="L %.1f, R %.1f, D %f", initial string=w446, w449, w450, w444) -> (resulting string=w445:string)  [unwired: 1 in, 1 out]
        "Current\nCmd" <- w445
        n222 = call <vilib>:"Trace Results.vi"("Status of previous command"=w451, "Description"=w445, "Subsystem"=w443) -> ()  [unwired: 9 in]
      }
    }
    n223 = call <vilib>:"WPI_RobotDriveMotors.vi"("RightSpeed"=w118, "LeftSpeed"=w119, "RobotDriveDevRef"=w124) -> ()  [unwired: 1 in, 8 out]
    n224 = call <vilib>:"WPI_RobotDriveMotors.vi"("RightSpeed"=w118, "LeftSpeed"=w119, "RobotDriveDevRef"=w123) -> ()  [unwired: 1 in, 8 out]
  }
  n225 = while {
    tunnel: w20 -> [w453]
    stop <- FALSE stop-if-true
    n226 = call "Drive Controller Interactive Check.vi"("Interactive Command In"="Interactive Values", "Default Command"=w453, "Buttons"="Buttons") -> ("Interactive Command Out"=w455:T3, "Trace String"=w456:string, "Schedule"=w457:bool)  [unwired: 6 in]
    n227 = case shown="False" w457 {
      tunnel: [w466 w474] -> w458
      tunnel: [w465 w470] -> w459
      tunnel: w456 -> [_ w472]
      tunnel: w455 -> [_ w471]
      frame False {
        n228 = Tick Count (ms)() -> (millisecond timer value=w469:u32)
        n229 = call "Read Drive Operation.vi"() -> ("Command Info"=w463:T25, "SubSystem Data"=w462:T3)  [unwired: 9 in, 1 out]
        n230 = Unbundle(w462) -> ("Operation"=w467:T4, "Left Speed"=w464:dbl)  [unwired: 9 out]
        n231 = Unbundle(w463) -> ("Status"=w466:T6)  [unwired: 2 out]
        n232 = Subtract(x=w469, y=w467) -> (x-y=w468:u32)
        n233 = Bundle(w468, "Left Speed"=w464) -> (w465:cluster{u32, "Left Speed":dbl})  [unwired: 1 in]
      }
      frame True {
        n234 = call "Drive Command Helper.vi"("Description"=w472, "SubSystem Data"=w471) -> ("Command Info Out"=w473:T25, "Command Timing"=w470:cluster{"Start Time (ms)":u32, "Iterations":i32})  [unwired: 7 in, 1 out]
        n235 = Unbundle(w473) -> ("Status"=w474:T6)  [unwired: 2 out]
      }
    }
    "Status" <- w458
    "Command Timing" <- w459
    n236 = Wait (ms)(milliseconds to wait=u32 20) -> ()  [unwired: 1 out]
  }
